vi "Test Compare I64 Cluster Data.vi"(11 "Cluster Assertion Test In":refnum<class "Cluster Assertion Test.lvclass">) -> (0 "error out":errorcluster, 3 "Cluster Assertion Test Out":refnum<class "Cluster Assertion Test.lvclass">)   [LabVIEW 2020, in "Cluster Assertion Test.lvclass"]
uses:
  Cluster Assertion Test.lvclass
  C:/Program Files (x86)/National Instruments/LabVIEW 2020/vi.lib/Astemes/LUnit/Test Case.lvclass
  source/LUnit Test Case.lvclass/LUnit Test Case.ctl
  <vilib>/Astemes/LUnit/Test Case.lvclass/Test Case.ctl
  2ac8ddb6-3846-4ca3-a318-916e2cedb3a3.vi
  06f0228f-1abf-4bd5-990f-da4968a7a7f9.vi
  1fc8a2ce-cd8f-4e65-8939-eca5f44e015b.vi
  source/Core/LUnit Test Case/Private/Append Pass Result.vi
  source/Core/LUnit Test Case/Private/Append Fail Result.vi
  2ac8ddb6-3846-4ca3-a318-916e2cedb3a3.vi/9c5d11cd-9439-4240-a1ee-d9baace9c924.vi
  06f0228f-1abf-4bd5-990f-da4968a7a7f9.vi/dc9e7da3-6f71-4ddf-bf72-545926b2b487.vi
  <vilib>/Astemes/LUnit/Core/LUnit Test Case/Private/Append Pass Result.vi
  <vilib>/Astemes/LUnit/Core/LUnit Test Case/Private/Append Fail Result.vi
  1fc8a2ce-cd8f-4e65-8939-eca5f44e015b.vi/9c5d11cd-9439-4240-a1ee-d9baace9c924.vi
  source/Core/LUnit Test Case/Private/Run In UI.vi
  06f0228f-1abf-4bd5-990f-da4968a7a7f9.vi/dc9e7da3-6f71-4ddf-bf72-545926b2b487.vi/9c5d11cd-9439-4240-a1ee-d9baace9c924.vi
  <vilib>/Astemes/LUnit/Core/LUnit Test Case/Private/Run In UI.vi
  <vilib>/Utility/error.llb/Clear Errors.vi
  <vilib>/Utility/LVClass/Get LV Class Name.vi
  source/Core/Advanced Assertions/Cluster to Array of Variants.vi
  source/LUnit Test Case.lvclass
  Cluster Assertion Test.lvclass/Cluster Assertion Test.ctl
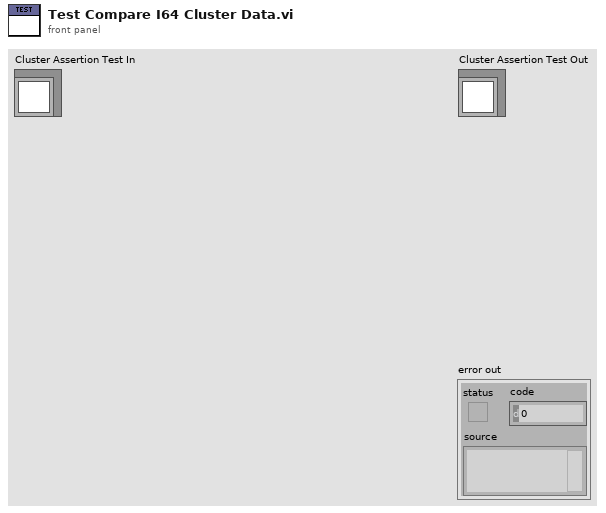
[diagram p1: front panel]
types:
  T1 = typedef "Result.lvlib/Result.ctl" = cluster{"Name":string, "Description":string, "Status":T2, "Result Type":T3, "Execution Time":dbl, "Data":cluster{"Expected":variant, "Actual":variant, "Delta":variant}}
  T2 = typedef "Result.lvlib/Status.ctl" = enum16{"", "Passed", "Failed", "Error", "Skipped", "Setup Error", "Broken", "Teardown Error"}
  T3 = typedef "Result.lvlib/Type.ctl" = enum16{"Test Case", "Test Suite", "Test Run", "Pass", "Fail", "Skip", "Pass if", "Fail if", "Pass if Error", "Fail if Error", "Pass if Equal", "Fail if Equal"}
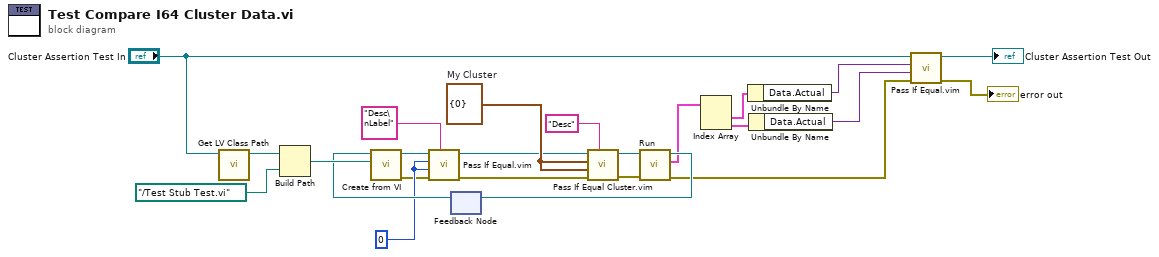
[diagram p0: block diagram]
diagram:
  w14 = i64 0
  w15 = cluster{"Label":i64} {"Label"=0}  # My Cluster
  n1 = call <vilib>:"Get LV Class Path.vi"("object"="Cluster Assertion Test In") -> ("class path"=w21:path)  [unwired: 9 in, 1 out]
  n2 = Build Path(base path=w21, name or relative path=path "../Test Stub Test.vi") -> (appended path=w19:path)
  n3 = feedback #1() -> (w18:refnum<class "LUnit Test Case.lvclass">)  [unwired: 1 in]
  n4 = call "Create from VI.vi"("Test Method VI Path"=w19, "LUnit Test Case In"=w18) -> ("error out"=w8:errorcluster, "LUnit Test Case Out"=w7:refnum<class "LUnit Test Case.lvclass">)  [unwired: 8 in]
  n5 = call "Pass If Equal.vim"("Description"="Desc\nLabel", "error in (no error)"=w8, "Actual"=w14, "Expected"=w14, "LUnit Test Case In"=w7) -> ("error out"=w4:errorcluster, "LUnit Test Case Out"=w6:refnum<class "LUnit Test Case.lvclass">)  [unwired: 5 in]
  n6 = call "Pass If Equal Cluster.vim"("Description"="Desc", "error in (no error)"=w4, "Actual Cluster"=w15, "Expected Cluster"=w15, "LUnit Test Case In"=w6) -> ("error out"=w3:errorcluster, "LUnit Test Case Out"=w5:refnum<class "LUnit Test Case.lvclass">)  [unwired: 5 in]
  n7 = call-dynamic "Run.vi"("error in (no error)"=w3, "LUnit Test Case In"=w5) -> ("error out"=w16:errorcluster, "Results"=w13:T1[], "LUnit Test Case Out"=w17:refnum<class "LUnit Test Case.lvclass">)  [unwired: 6 in, 1 out]
  n8 = feedback-in #1(w17) -> ()
  n9 = Index Array(array=w13) -> (element #1=w12:T1, element #2=w11:T1)  [unwired: 2 in]
  n10 = Unbundle By Name(w12) -> ("Data.Actual"=w9:variant)
  n11 = Unbundle By Name(w11) -> ("Data.Actual"=w10:variant)
  n12 = call "Pass If Equal.vim"("error in (no error)"=w16, "Actual"=w10, "Expected"=w9, "LUnit Test Case In"="Cluster Assertion Test In") -> ("error out"=→"error out":errorcluster, "LUnit Test Case Out"=→"Cluster Assertion Test Out":refnum<class "Cluster Assertion Test.lvclass">)  [unwired: 6 in]
